vi "Test Panel - Copy.vi"(8 "error in (no error)":errorcluster, 11 "VISA resource name":refnum<visa-resource-name>="COM3") -> (0 "error out":errorcluster, 3 "VISA resource name out":refnum<visa-resource-name>)   [LabVIEW 2017]
panel:
  in  "milliseconds to wait":u32
  out "PEM Name":string
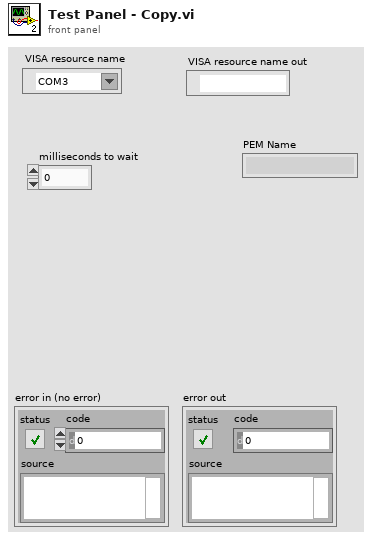
[diagram p1: front panel]
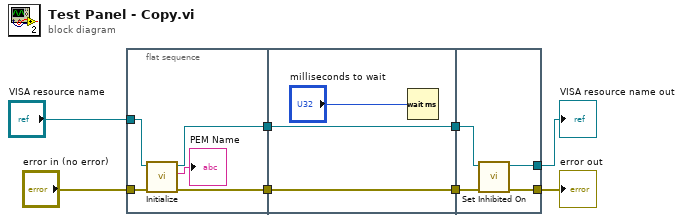
[diagram p0: block diagram]
diagram:
  n1 = flat-sequence {
    tunnel: "VISA resource name" -> [w13]
    tunnel: "error in (no error)" -> [w12]
    tunnel: [w10] -> w6
    tunnel: [w9] -> w5
    tunnel: w6 -> [w16]
    tunnel: w5 -> [w15]
    tunnel: [w16] -> w4
    tunnel: [w15] -> w3
    tunnel: w4 -> [w19]
    tunnel: w3 -> [w20]
    tunnel: [w18] -> w2
    tunnel: [w17] -> w1
    frame #0 {
      n2 = call "Initialize.vi"("error in (no error)"=w12, "VISA resource name"=w13) -> ("error out"=w9:errorcluster, "PEM Name"=→"PEM Name":string, "VISA resource name out"=w10:refnum<visa-resource-name>)  [unwired: 7 in]
    }
    frame #1 {
      n3 = Wait (ms)(milliseconds to wait="milliseconds to wait") -> ()  [unwired: 1 out]
    }
    frame #2 {
      n4 = call "Set Inhibited On.vi"("error in (no error)"=w20, "VISA resource name"=w19) -> ("error out"=w18:errorcluster, "VISA resource name out"=w17:refnum<visa-resource-name>)  [unwired: 7 in, 1 out]
    }
  }
  "error out" <- w2
  "VISA resource name out" <- w1
